vi "Reset XNET.vi"(8 "error in (no error)":errorcluster) -> (0 "error out":errorcluster)   [LabVIEW 2019, in "Reset Hardware Engine.lvlib"]
uses:
  <vilib>/DAQmx/miscellaneous.llb/DAQmx Fill In Error Info.vi
  Reset Hardware Engine.lvlib
  <resource>/objmgr/nicontrollersysapi.rc
  <vilib>/nisyscfg/nisyscfg.lvlib
  <vilib>/NI VeriStand/Custom Device Tools/Custom Device Utility Library/Custom Device Utility Library.lvlib
  <resource>/objmgr/niflexrioatomicsae.rc
  <vilib>/nisyscfg/Close (System).vi
  <vilib>/nisyscfg/Close (Filter).vi
  <vilib>/nisyscfg/Close (Hardware).vi
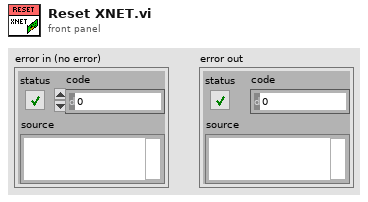
[diagram p1: front panel]
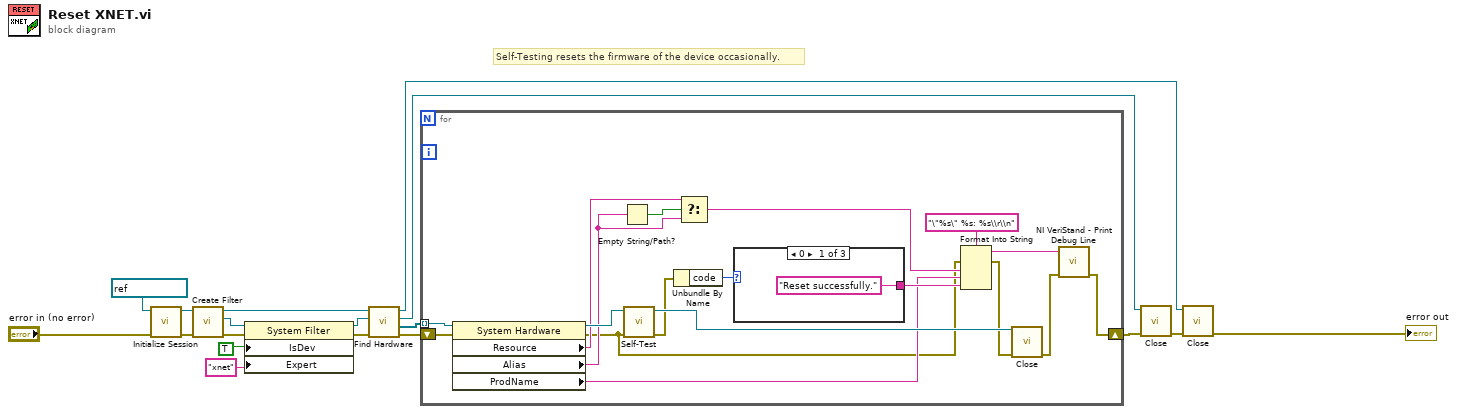
[diagram p0: block diagram]
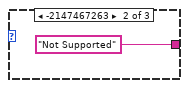
[diagram p2: hidden frame]
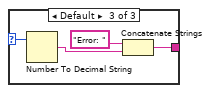
[diagram p3: hidden frame]
diagram:
  # "Self-Testing resets the firmware of the device occasionally."
  n1 = call <vilib>:"Initialize Session.vi"("error in (no error)"="error in (no error)", "Target (localhost)"=refnum<k21> "localhost") -> ("error out"=w7:errorcluster, "Session out"=w6:refnum<k21>)  [unwired: 8 in]
  n2 = call <vilib>:"Create Filter.vi"("error in (no error)"=w7, "Session in"=w6) -> ("error out"=w11:errorcluster, "Filter out"=w8:refnum<k20>, "Session out"=w5:refnum<k21>)  [unwired: 7 in]
  n3 = property class="System Filter"(reference=w8, error in=w11, "IsDev"=TRUE ("Is Device"), "Expert"="xnet" ("Expert Info:Expert Name")) -> (reference out=w9:refnum<k20>, error out=w12:errorcluster)
  n4 = call <vilib>:"Find Hardware.vi"("error in (no error)"=w12, "Filter in"=w9, "Session in"=w5) -> ("error out"=w4:errorcluster, "Resources out"=w3:refnum<k20>[], "Filter out"=w15:refnum<k20>, "Session out"=w16:refnum<k21>)  [unwired: 1 in, 4 out]
  n5 = for {
    tunnel: w3 -> [w35] mode=indexing
    shift-right: [w20] -> w14
    shift-left: w4 -> [w34]
    n6 = property class="System Hardware"(reference=w35, error in=w34) -> (reference out=w33:refnum<k20>, error out=w23:errorcluster, "Resource"=w29:string, "Alias"=w28:string, "ProdName"=w25:string)
    n7 = Empty String/Path?(string/path=w28) -> (empty?=w36:bool)
    n8 = call <vilib>:"Self-Test.vi"("error in (no error)"=w23, "Resource in"=w33) -> ("error out"=w30:errorcluster, "Resource out"=w32:refnum<k20>)  [unwired: 7 in, 1 out]
    n9 = Unbundle By Name(w30) -> ("code"=w31:i32)
    n10 = Select(t=w29, s=w36, f=w28) -> (s? t:f=w24:string)
    n11 = case shown="0" w31 {
      selector: w31 -> [_ _ w40]
      tunnel: ["Reset successfully." ("L10n_Pass") "Not Supported" ("L10n_NotSupported") w39] -> w26
      frame 0 {
      }
      frame -2147467263 {
      }
      frame Default {
        n12 = Number To Decimal String(number=w40) -> (decimal integer string=w42:string)  [unwired: 1 in]
        n13 = Concatenate Strings("Error: " ("L10n_Error"), w42) -> (w39:string)
      }
    }
    n14 = Format Into String(format string="\"%s\" %s: %s\\r\\n", error in=w23, w24, w25, w26) -> (resulting string=w19:string, error out=w22:errorcluster)  [unwired: 1 in]
    n15 = call-poly <vilib>:"Close.vi"("error in (no error)"=w22, "Resource in"=w32) -> ("error out"=w21:errorcluster)  [unwired: 9 in]
    n16 = call <vilib>:"NI VeriStand - Print Debug Line.vi"("error in (no error)"=w21, "Message"=w19) -> ("error out"=w20:errorcluster)  [unwired: 9 in]
  }
  n17 = call-poly <vilib>:"Close.vi"("error in (no error)"=w14, "Filter in"=w15) -> ("error out"=w13:errorcluster)  [unwired: 9 in]
  n18 = call-poly <vilib>:"Close.vi"("error in (no error)"=w13, "Session in"=w16) -> ("error out"=→"error out":errorcluster)  [unwired: 9 in]
